vi "Set Position.vi"(8 "error in (no error)":errorcluster, 10 "Position":dbl, 11 "Servo Motor Emulator in":refnum<class "Servo Motor Emulator.lvclass">) -> (0 "error out":errorcluster, 3 "Servo Motor Emulator out":refnum<class "Servo Motor Emulator.lvclass">)   [LabVIEW 2020, in "Servo Motor Emulator.lvlib" / "Servo Motor Emulator.lvclass"]
uses:
  Servo Motor Emulator.lvclass
  Servo Motor Emulator.lvclass/Servo Motor Emulator.ctl
  Panel/Panel Messages/Report Actual Position Msg/Report Actual Position Msg.lvclass
  <vilib>/ActorFramework/Actor/Actor.lvclass
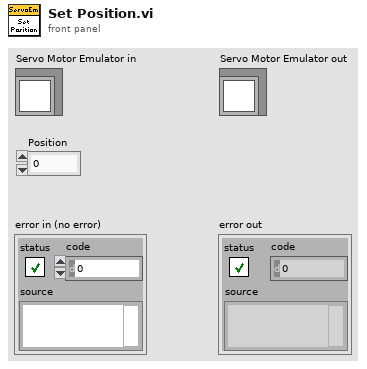
[diagram p1: front panel]
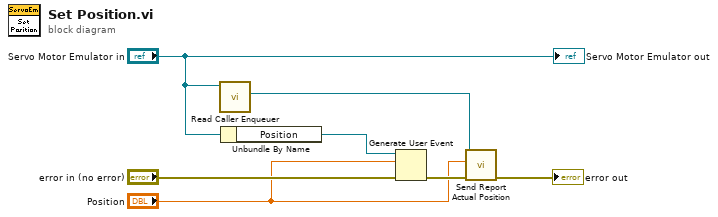
[diagram p0: block diagram]
diagram:
  n1 = call <vilib>:"Read Caller Enqueuer.vi"("Actor"="Servo Motor Emulator in") -> ("Caller Enqueuer"=w3:refnum<class "Message Enqueuer.lvclass">)  [unwired: 10 in]
  n2 = Unbundle By Name("Servo Motor Emulator in") -> ("Position"=w7:refnum<user-event>)
  n3 = Generate User Event(user event=w7, event data cluster="Position", error in="error in (no error)") -> (error out=w4:errorcluster)  [unwired: 1 in, 1 out]
  n4 = call "Send Report Actual Position.vi"("error in (no error)"=w4, "Actual Position"="Position", "Message Enqueuer"=w3) -> ("error out"=→"error out":errorcluster)  [unwired: 7 in, 1 out]
  "Servo Motor Emulator out" <- "Servo Motor Emulator in"
